vi "WinDebugLogging.vi"(4 "message":string, 6 "error in (no error)":errorcluster, 7 "prefix":string="LVDebug") -> (1 "error out":errorcluster)   [LabVIEW 2014]
uses:
  kernel32.dll
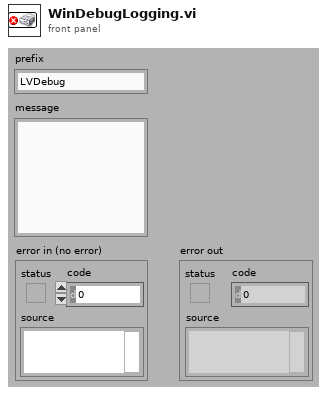
[diagram p1: front panel]
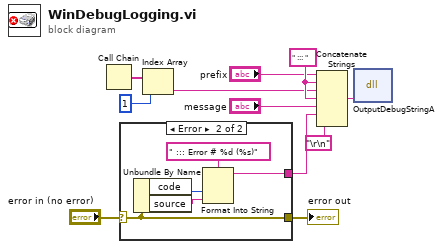
[diagram p0: block diagram]
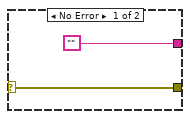
[diagram p2: hidden frame]
diagram:
  w3 = " ::: "
  n1 = Call Chain() -> (call chain=w11:string[])
  n2 = case shown="Error" "error in (no error)" {
    selector: "error in (no error)" -> [w13 w17]
    tunnel: [w13 w17] -> w6
    tunnel: ["" w14] -> w5
    frame No Error {
    }
    frame Error {
      n3 = Unbundle By Name(w17) -> ("code"=w15:i32, "source"=w16:string)
      n4 = Format Into String(format string=" ::: Error # %d (%s)", w15, w16) -> (resulting string=w14:string)  [unwired: 2 in, 1 out]
    }
  }
  "error out" <- w6
  n5 = Index Array(array=w11, index=1) -> (element=w2:string)
  n6 = Concatenate Strings("prefix", w3, w2, w3, "message", w5, "\r\n") -> (w9:string)
  n7 = dll-call lib="Kernel32.dll" fn="OutputDebugStringA"("debugString"=w9) -> ()  [unwired: 5 in, 2 out]
